vi "Choose Tank.vi"() -> (2 "Device":T1[](array[typedef]))   [LabVIEW 2011]
uses:
  Valve_Pump.ctl
  Pumps_Valves_Dependencies_Global.vi
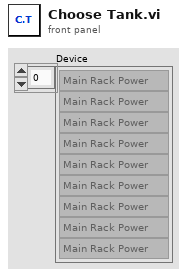
[diagram p1: front panel]
types:
  T1 = typedef "Valve_Pump.ctl" = enum16{"Main Rack Power", "Pump Power", "Valve Power", "V4", "V5", "V6", "V7", "V8", "V9", "V10", "V11", "V12", "V13", "V14", "V15", "V18", "V19", "V20", "V21", "V22", "V23", "V24", "V25", "V26", "V27", "V28", "V29", "V30", "V31", "V32", "V33", "V34", "Pump A", "Pump B", "Pump C", "Pump D"}
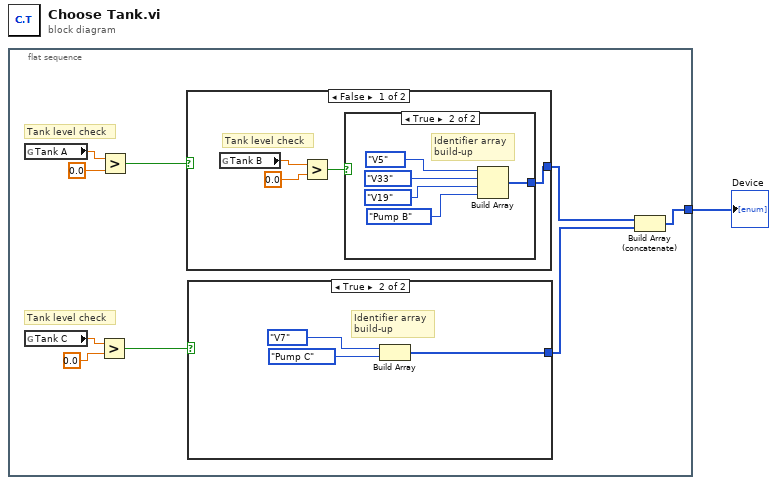
[diagram p0: block diagram]
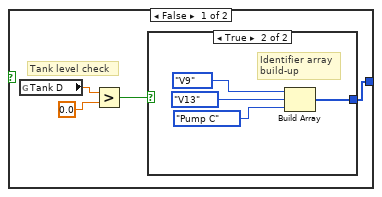
[diagram p2: hidden frame]
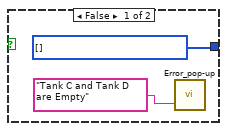
[diagram p3: hidden frame]
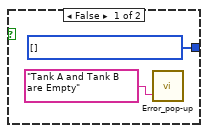
[diagram p4: hidden frame]
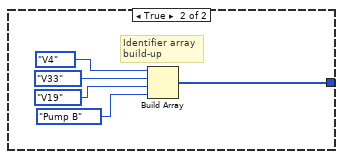
[diagram p5: hidden frame]
diagram:
  n1 = flat-sequence {
    tunnel: [w10] -> w1
    frame #0 {
      # "Tank level check"
      # "Tank level check"
      n2 = global read "Pumps_Valves_Dependencies_Global.vi" "Tank A"() -> (w7:dbl)
      n3 = global read "Pumps_Valves_Dependencies_Global.vi" "Tank C"() -> (w8:dbl)
      n4 = Greater?(x=w8, y=0.0) -> (0:w9:bool)
      n5 = Greater?(x=w7, y=0.0) -> (0:w4:bool)
      n6 = case shown="False" w4 {
        tunnel: [w24 w35] -> w3
        frame False {
          # "Tank level check"
          n7 = global read "Pumps_Valves_Dependencies_Global.vi" "Tank B"() -> (w27:dbl)
          n8 = Greater?(x=w27, y=0.0) -> (0:w25:bool)
          n9 = case shown="True" w25 {
            tunnel: [w28 w30] -> w24
            frame False {
              w28 = T1[] [] items=["Main Rack Power", "Pump Power", "Valve Power", "V4", "V5", "V6", "V7", "V8", "V9", "V10", "V11", "V12", "V13", "V14", "V15", "V18", "V19", "V20", "V21", "V22", "V23", "V24", "V25", "V26", "V27", "V28", "V29", "V30", "V31", "V32", "V33", "V34", "Pump A", "Pump B", "Pump C", "Pump D"]
              n10 = call "Error_pop-up.vi"("New msg"="Tank A and Tank B are Empty") -> ()  [unwired: 2 in]
            }
            frame True {
              # "Identifier array\nbuild-up"
              n11 = Build Array(Valve_Pump."V5" ("Device"), Valve_Pump."V33" ("Device"), Valve_Pump."V19" ("Device"), Valve_Pump."Pump B" ("Device")) -> (w30:T1[])
            }
          }
        }
        frame True {
          # "Identifier array\nbuild-up"
          n12 = Build Array(Valve_Pump."V4" ("Device"), Valve_Pump."V33" ("Device"), Valve_Pump."V19" ("Device"), Valve_Pump."Pump B" ("Device")) -> (w35:T1[])
        }
      }
      n13 = case shown="True" w9 {
        tunnel: [w11 w21] -> w2
        frame False {
          # "Tank level check"
          n14 = global read "Pumps_Valves_Dependencies_Global.vi" "Tank D"() -> (w14:dbl)
          n15 = Greater?(x=w14, y=0.0) -> (0:w12:bool)
          n16 = case shown="True" w12 {
            tunnel: [w15 w17] -> w11
            frame False {
              w15 = T1[] [] items=["Main Rack Power", "Pump Power", "Valve Power", "V4", "V5", "V6", "V7", "V8", "V9", "V10", "V11", "V12", "V13", "V14", "V15", "V18", "V19", "V20", "V21", "V22", "V23", "V24", "V25", "V26", "V27", "V28", "V29", "V30", "V31", "V32", "V33", "V34", "Pump A", "Pump B", "Pump C", "Pump D"]
              n17 = call "Error_pop-up.vi"("New msg"="Tank C and Tank D are Empty") -> ()  [unwired: 2 in]
            }
            frame True {
              # "Identifier array\nbuild-up"
              n18 = Build Array(Valve_Pump."V9" ("Device"), Valve_Pump."V13" ("Device"), Valve_Pump."Pump C" ("Device")) -> (w17:T1[])
            }
          }
        }
        frame True {
          # "Identifier array\nbuild-up"
          n19 = Build Array(Valve_Pump."V7" ("Device"), Valve_Pump."Pump C" ("Device")) -> (w21:T1[])
        }
      }
      n20 = Build Array (concatenate)(w3, w2) -> (w10:T1[])
    }
  }
  "Device" <- w1
